vi "Write_Read.vi"(7 "delay before read (ms)":u32=100, 8 "error in (no error)":errorcluster, 10 "String":string, 11 "VISA Refnum in":refnum<visa-resource-name>) -> (0 "error out":errorcluster, 2 "Response":string, 3 "VISA resource name out":refnum<visa-resource-name>)   [LabVIEW 2024]
doc: "Write a command and read the response from the device"
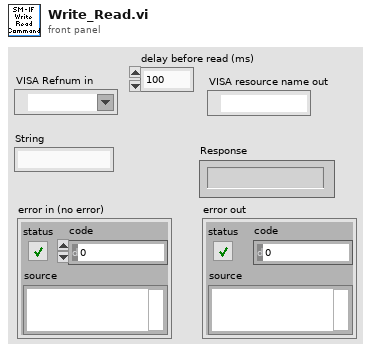
[diagram p1: front panel]
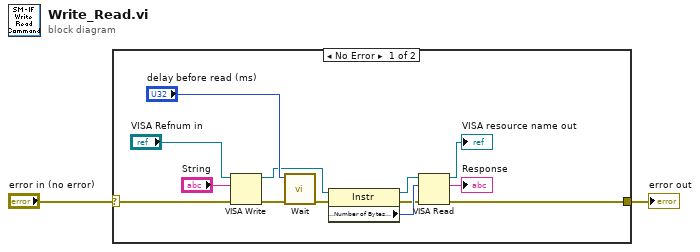
[diagram p0: block diagram]
diagram:
  n1 = case shown="No Error" "error in (no error)" {
    selector: "error in (no error)" -> [w8 w16]
    tunnel: [w14 w16] -> w2
    frame No Error {
      n2 = VISA Write(VISA resource name="VISA Refnum in", write buffer="String", error in (no error)=w8) -> (VISA resource name out=w3:refnum<visa-resource-name>, error out=w5:errorcluster)  [unwired: 1 out]
      n3 = call "Wait.vi"("error in (no error)"=w5, "milliseconds to wait"="delay before read (ms)") -> ("error out"=w4:errorcluster)  [unwired: 9 in]
      n4 = property class="Instr"(reference=w3, error in=w4) -> (reference out=w10:refnum<visa-resource-name>, error out=w11:errorcluster, "Serial Settings:Number of Bytes at Serial Port"=w13:u32)
      n5 = VISA Read(VISA resource name=w10, byte count=w13, error in (no error)=w11) -> (VISA resource name out=→"VISA resource name out":refnum<visa-resource-name>, read buffer=→"Response":string, error out=w14:errorcluster)  [unwired: 1 out]
    }
    frame Error {
    }
  }
  "error out" <- w2
